vi "PushingState.vi"(8 "error in (no error)":errorcluster, 9 "Cluster in":T2, 10 "Enum in":T1, 11 "Actual Start [i]":i64) -> (0 "error out":errorcluster, 2 "Cluster out":T2, 3 "Enum":T1)   [LabVIEW 2018]
uses:
  Type_Def/Type_Def Actuator Controls.ctl
  Type_Def/Type_Def ControlState.ctl
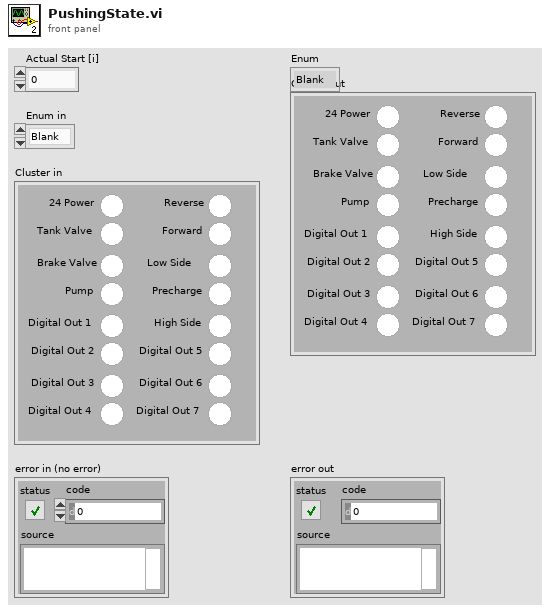
[diagram p1: front panel]
types:
  T1 = typedef "Type_Def ControlState.ctl" = enum16{"Blank", "Systems Check", "Idle", "Ready", "Pushing", "CrawlingPrecharge", "Braking", "Fault", "Boot Up", "Unpowered", "Crawling", "Shutdown", "Service Push", "Service Wait", "Vent", "Precharge", "Cooldown"}
  T2 = typedef "Type_Def Actuator Controls.ctl" = cluster{"Reverse ":bool, "Forward":bool, "Low Side":bool, "Precharge":bool, "High Side":bool, "Digital Out 5":bool, "Digital Out 6":bool, "Digital Out 7 ":bool, "24 Power":bool, "Tank Valve ":bool, "Brake Valve":bool, "Pump":bool, "Digital Out 1 ":bool, "Digital Out 2":bool, "Digital Out 3":bool, "Digital Out 4 ":bool}
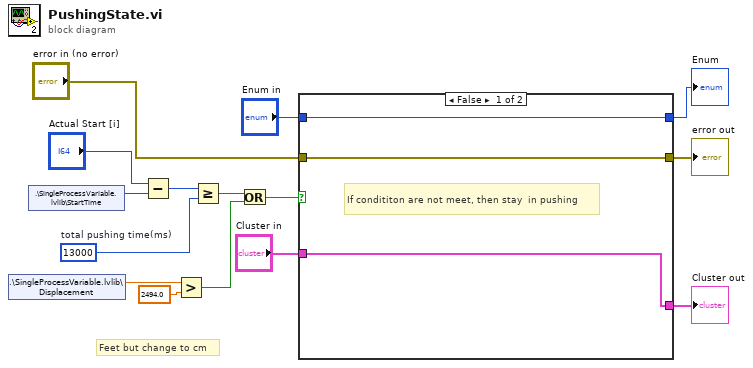
[diagram p0: block diagram]
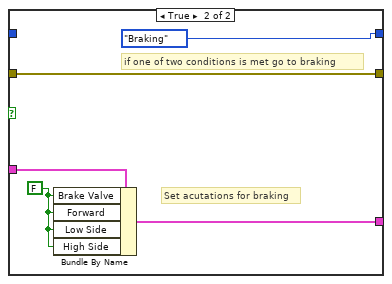
[diagram p2: hidden frame]
diagram:
  w10 = i64 13000  # total pushing time(ms)
  # "Feet but change to cm"
  n1 = shared-variable ".\\SingleProcessVariable.lvlib\\Displacement"() -> (w15:dbl)  [unwired: 1 in, 1 out]
  n2 = shared-variable ".\\SingleProcessVariable.lvlib\\StartTime"() -> (w8:i64)  [unwired: 1 in, 1 out]
  n3 = Subtract(x="Actual Start [i]", y=w8) -> (x-y=w9:i64)
  n4 = Greater?(x=w15, y=2494.0 ("Feet but change to cm")) -> (0:w14:bool)
  n5 = Greater Or Equal?(x=w9, y=w10) -> (x >= y?=w11:bool)
  n6 = Or(x=w11, y=w14) -> (x .or. y?=w12:bool)
  n7 = case shown="False" w12 {
    tunnel: "Enum in" -> [w18 _]
    tunnel: [w18 Type_Def_ControlState."Braking"] -> w2
    tunnel: "Cluster in" -> [w17 w22]
    tunnel: [w17 w21] -> w4
    tunnel: [w16 w20] -> w5
    tunnel: "error in (no error)" -> [w16 w20]
    frame False {
      # "If condititon are not meet, then stay  in pushing"
    }
    frame True {
      w19 = FALSE ("Digital Out 5")
      # "Set acutations for braking"
      # "if one of two conditions is met go to braking"
      n8 = Bundle By Name(cluster=w22, "Brake Valve"=w19, "Forward"=w19, "Low Side"=w19, "High Side"=w19) -> (w21:T2)
    }
  }
  "error out" <- w5
  "Cluster out" <- w4
  "Enum" <- w2
